vi "CSM - Mark As System-Level Module.vi"(9 "CSM Name":string) -> (2 "CSM Name (Marked As Sysetem-Level Module)":string)   [LabVIEW 2017, in "Communicable State Machine.lvlib"]
doc: "Marks a module as a system-level module by adding `.` before the input string. For example, if the input is `UIModule`, the output is `.UIModule`.\n\n<b>Reference Example</b>: `0. Base Concepts\\7. System-Level Module.vi`.\n\n\n> [!NOTE] <b>Name Concatenation API</b>\n>\n> This VI only manipulates the module name string and has no actual functionality. Therefore, once you are familiar with the CSM rules, you can directly enter name string and rule symbols without calling this API.\n\n\n> [!NOTE] <b>CSM System-Level Module</b>\n>\n> CSM functions of a system-level module are almost identical to those of a normal module. The only difference is that the CSM - List Modules VI does not list system-level modules. Therefore, a system-level module is typically used to implement functional modules running in the background. When processing the operational logic of normal modules in a unified manner, interference with these background running logics can be avoided.\n>\n> CSM system-level modules usually start with `.`, for example: `.MainApp` and `.BackgroundTask`. The `.` is part of the name, so operations like message sending and registration must include the `.` in the name. For example, you can name the main program loop `.MainApp`. You can then use the CSM - List Modules VI to get a list of all normal modules without listing `.MainApp`. If the main program needs to exit all other modules, you can send \"Macro: Exit\" to the results of the CSM - List Modules VI. This allows you to exit all normal modules without affecting the operation of the system-level module.\n>\n> CSM modules in Worker Mode and Chain of Responsibility Mode can also start with `.` and run as system-level modules.\n\n\n-- <b>Controls</b> --\n- <b>CSM Name</b>: CSM module name.\n\n-- <b>Indicators</b> --\n- <b>CSM Name (Marked As System-Level Module)</b>: CSM module name marked with `.`."
uses:
  Communicable State Machine.lvlib
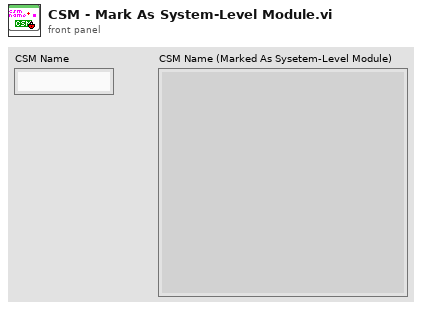
[diagram p1: front panel]
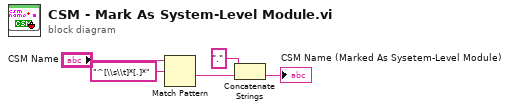
[diagram p0: block diagram]
diagram:
  n1 = Match Pattern(string="CSM Name", regular expression="^[\\s\\t]*[.]*") -> (after substring=w1:string)  [unwired: 1 in, 3 out]
  n2 = Concatenate Strings("." ("string"), w1) -> (→"CSM Name (Marked As Sysetem-Level Module)":string)
